vi "Dialog GraphSetting (Wave).vi"(11 "波形グラフref(in)":refnum<vi>) -> ()   [LabVIEW 2014]
uses:
  TypeDef/GraphSetting Appearance.ctl
  TypeDef/GraphSetting Plot.ctl
  SupportVIs/GraphSetting Scale.ctl
  TypeDef/GraphSetting DisplayFormatType.ctl
  TypeDef/GraphSetting All.ctl
  TypeDef/GraphSetting Command.ctl
  Lib/Event/Write User Event (Array).vi
  <vilib>/Utility/xml.llb/Write to XML File(string).vi
  <vilib>/Utility/xml.llb/Read From XML File(string).vi
  <vilib>/measure/NI_MABase.lvlib
panel:
  out "波形グラフ":cluster{dbl, "dt":dbl, "Y":dbl[]}[](graph)
  in  "ファイル読込":bool
  in  "ファイル保存":bool
  in  "タブ制御器":enum32{"外観", "スケール", "プロット"}(tab)
  in  "外観":T1
  in  "Yスケール選択":u16(ring) items=["振幅"]
  in  "スケール(Y軸)":T2
  in  "スケール(X軸)":T2
  in  "Xスケール選択":u16(ring) items=["周波数"]
  in  "プロット":T4 {"Yスケール" items=["振幅"]; "Xスケール" items=["周波数"]; "プロット補間" max=5 step=1; "ポイントスタイル" max=16 step=1; "太さ" max=5 step=1; "ラインスタイル" max=4 step=1}
  in  "プロット選択":u16(ring) items=["プロット0", "プロット1"]
  in  "停止ボタン":bool
  # "スケールのスタイルとカラー"
  # "スケール係数"
  # "スケールのスタイルとカラー"
  # "スケールのスタイルとカラー"
  # "スケール係数"
  # "スケールのスタイルとカラー"
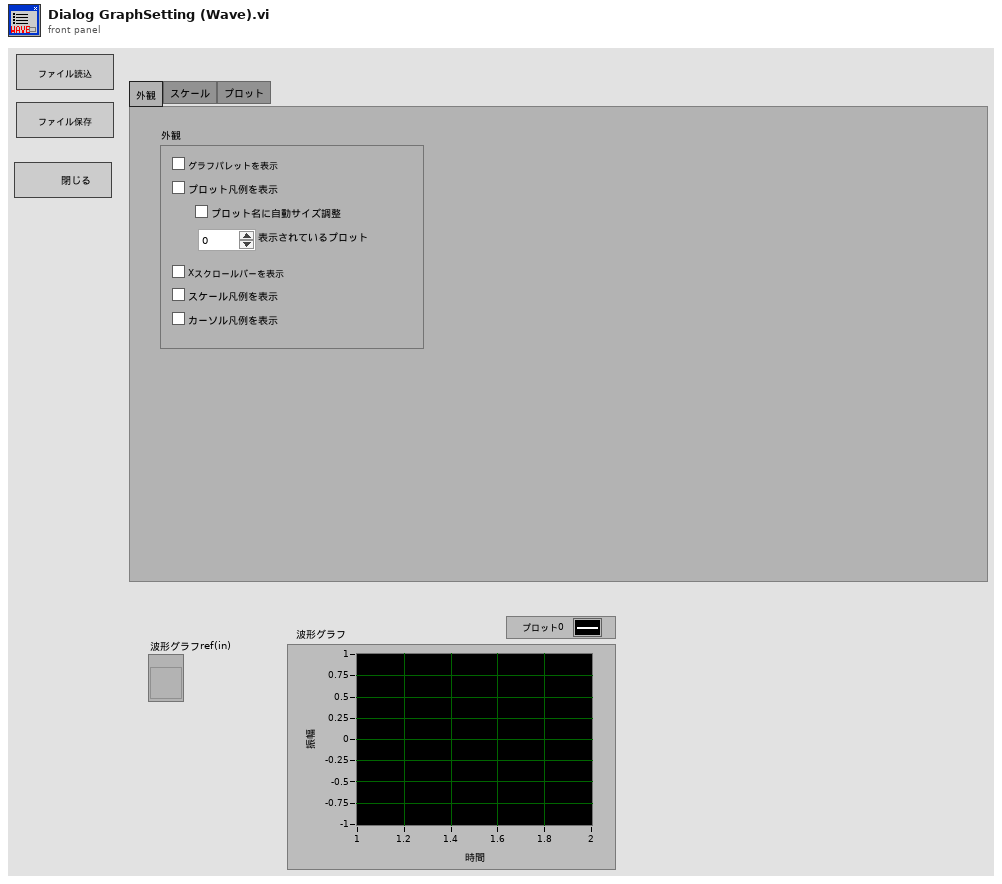
[diagram p1: front panel]
types:
  T1 = typedef "GraphSetting Appearance.ctl" = cluster{"グラフパレットを表示":bool, "プロット凡例を表示":bool, "プロット名に自動サイズ調整":bool, "表示されているプロット":u32, "Xスクロールバーを表示":bool, "スケール凡例を表示":bool, "カーソル凡例を表示":bool}
  T2 = typedef "GraphSetting Scale.ctl" = cluster{"名前":string, "スケールラベルを表示":bool, "スケールを表示":bool, "ログ":bool, "反転":bool, "自動スケール":bool, "最小":dbl, "最大":dbl, "オフセット":dbl, "乗数":dbl, "主目盛り":u32, "補助目盛り":u32, "マーカテキスト":u32, "主グリッド":u32, "補助グリッド":u32, "タイプ":T3, "小数点以下桁数":u8}
  T3 = typedef "GraphSetting DisplayFormatType.ctl" = enum8{"浮動小数点", "科学", "工学", "バイナリ", "８進数", "１６進数", "相対時間", "時間と日時", "SI"}
  T4 = typedef "GraphSetting Plot.ctl" = cluster{"名前":string, "表示":bool, "ラインスタイル":u8, "太さ":u8, "ポイントスタイル":u8, "プロット補間":u8, "ラインカラー":u32, "ポイント/塗りつぶし":u32, "Xスケール":u16, "Yスケール":u16}
  T5 = typedef "GraphSetting All.ctl" = cluster{"外観":T1, "スケールX[]":T2[], "スケールY[]":T2[], "プロット[]":T4[]}
  T6 = typedef "GraphSetting Command.ctl" = enum16{"Get(ref->ctl)", "Set(ctl->ref)"}
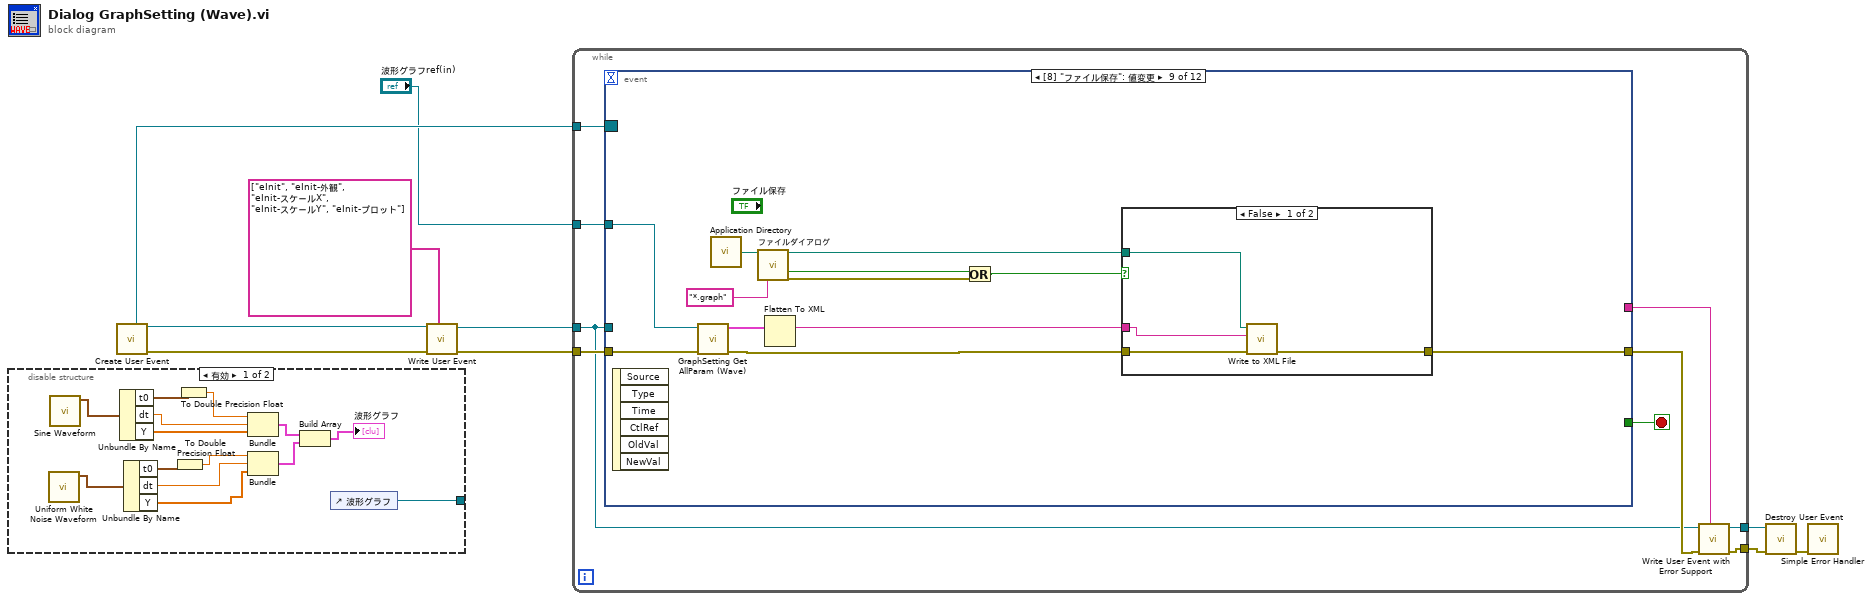
[diagram p0: block diagram]
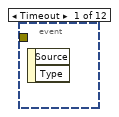
[diagram p3: hidden frame]
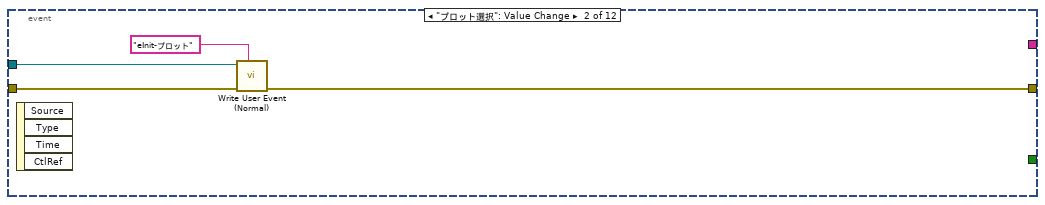
[diagram p4: hidden frame]
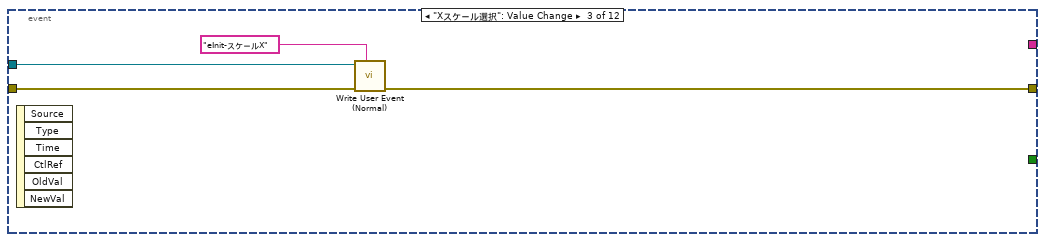
[diagram p5: hidden frame]
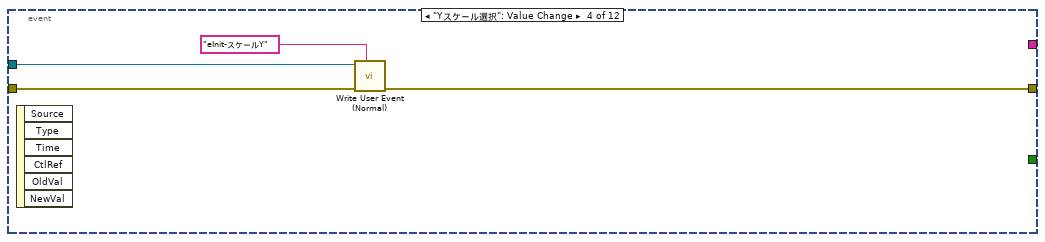
[diagram p6: hidden frame]
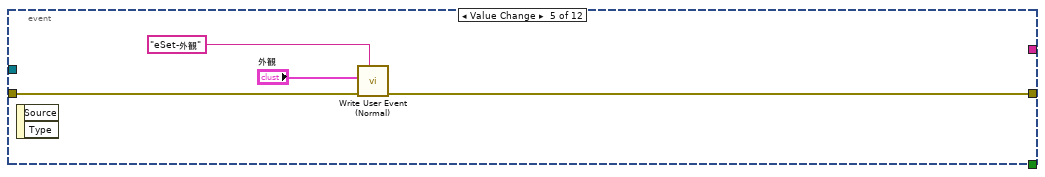
[diagram p7: hidden frame]
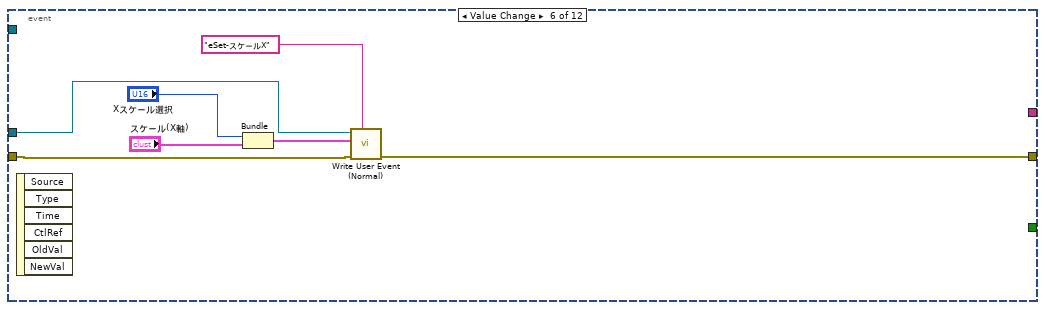
[diagram p8: hidden frame]
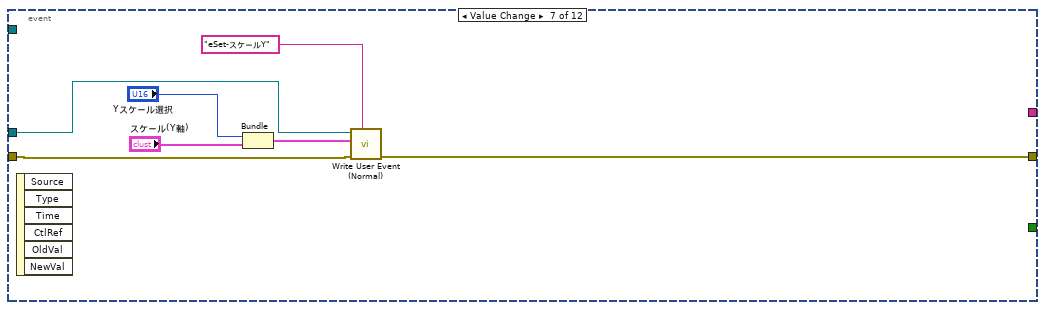
[diagram p9: hidden frame]
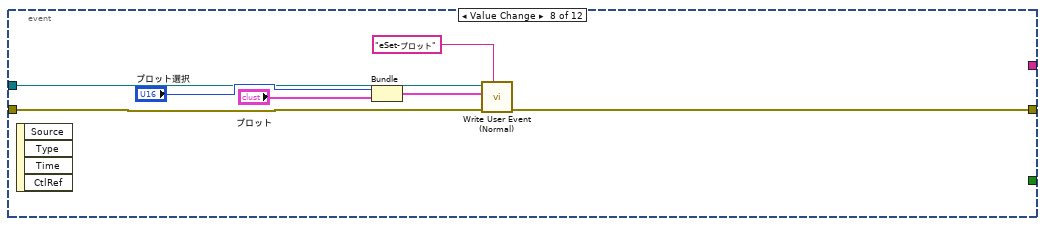
[diagram p10: hidden frame]
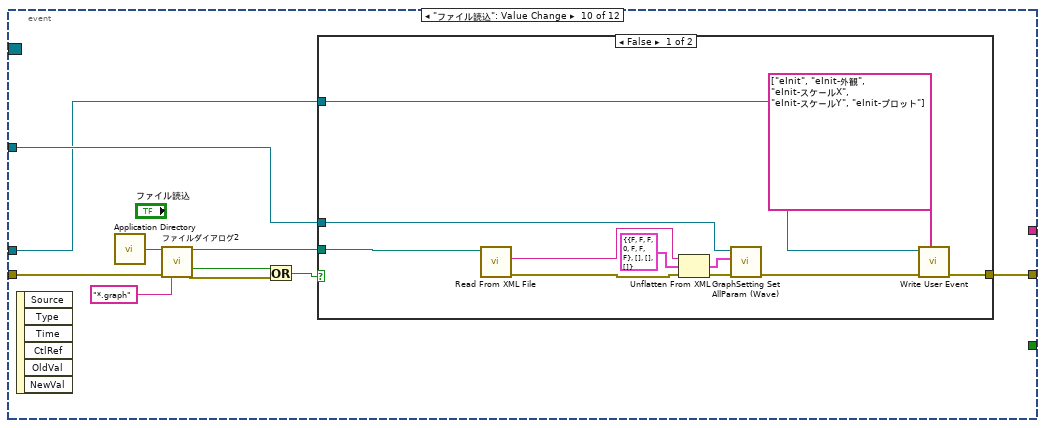
[diagram p12: hidden frame]
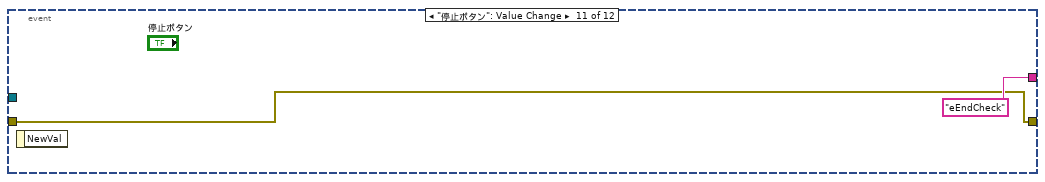
[diagram p14: hidden frame]
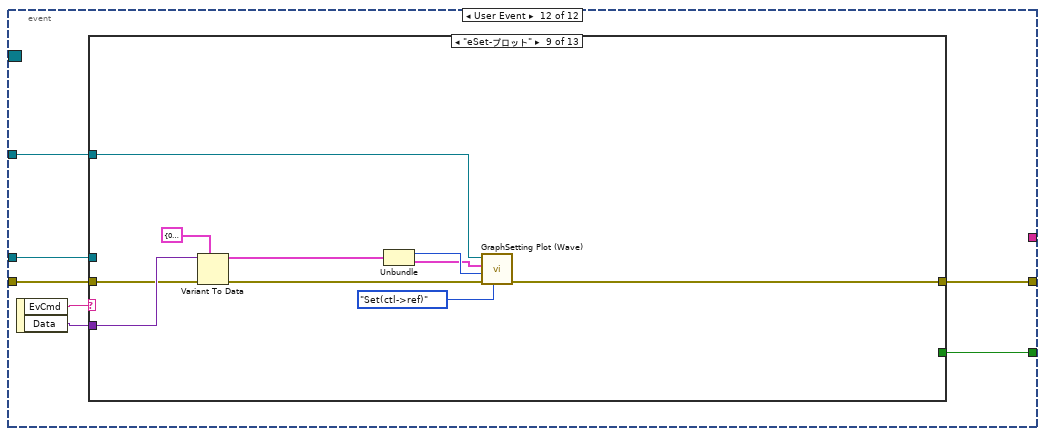
[diagram p15: hidden frame]
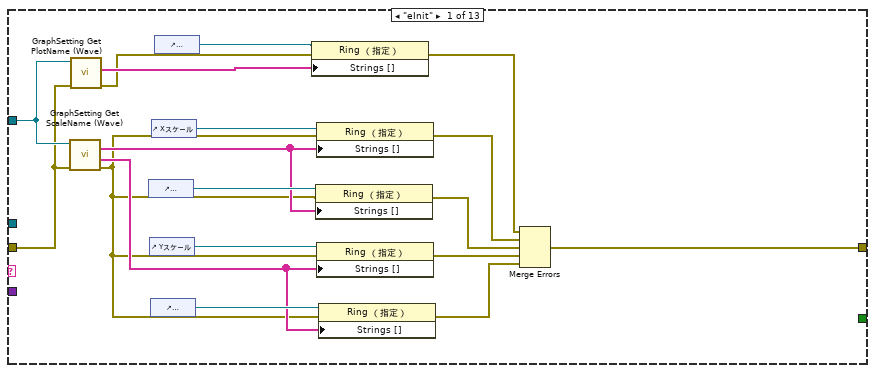
[diagram p16: hidden frame]
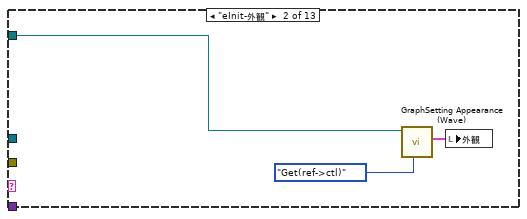
[diagram p17: hidden frame]
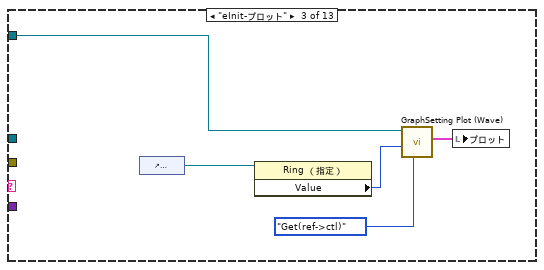
[diagram p18: hidden frame]
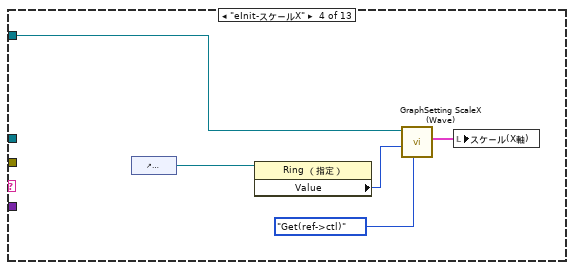
[diagram p19: hidden frame]
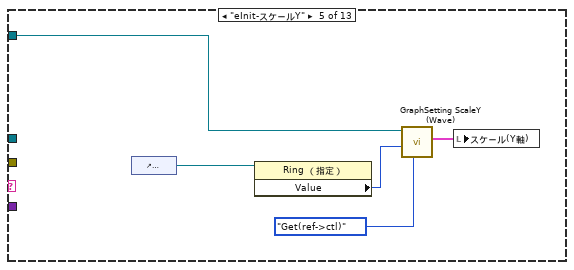
[diagram p20: hidden frame]
diagram:
  n1 = disable-structure shown="有効" {
    disable-tunnel: [w11 _] -> _
    frame Enabled {
      n2 = call <vilib>:"Uniform White Noise Waveform.vi"() -> ("signal out"=w19:waveform(dbl))  [unwired: 10 in, 1 out]
      n3 = call <vilib>:"Sine Waveform.vi"() -> ("signal out"=w24:waveform(dbl))  [unwired: 10 in, 1 out]
      n4 = Unbundle By Name(w24) -> ("t0"=w23:timestamp, "dt"=w21:dbl, "Y"=w20:dbl[])
      n5 = Unbundle By Name(w19) -> ("t0"=w18:timestamp, "dt"=w16:dbl, "Y"=w15:dbl[])
      n6 = To Double Precision Float(number=w18) -> (double precision float=w17:dbl)
      n7 = To Double Precision Float(number=w23) -> (double precision float=w22:dbl)
      n8 = Bundle(w22, "dt"=w21, "Y"=w20) -> (w14:cluster{dbl, "dt":dbl, "Y":dbl[]})  [unwired: 1 in]
      n9 = Bundle(w17, "dt"=w16, "Y"=w15) -> (w13:cluster{dbl, "dt":dbl, "Y":dbl[]})  [unwired: 1 in]
      n10 = Build Array(w14, w13) -> (→"波形グラフ":cluster{dbl, "dt":dbl, "Y":dbl[]}[])
      n11 = control-ref of="波形グラフ"() -> (w11:refnum<vi>)
    }
    frame Disabled {
    }
  }
  n12 = call "Create User Event.vi"() -> ("error out"=w8:errorcluster, "User Event"=w9:refnum<user-event>, "Event Registration Refnum"=w10:refnum<event-registration>)  [unwired: 9 in]
  n13 = call-poly "Write User Event.vi"("EvCmd[]"=string[] ["eInit", "eInit-外観", "eInit-スケールX", "eInit-スケールY", "eInit-プロット"], "エラー入力（エラーなし）"=w8, "ユーザイベント入力"=w9) -> ("エラー出力"=w4:errorcluster, "ユーザイベント出力"=w5:refnum<user-event>)  [unwired: 7 in]
  n14 = while {
    tunnel: w4 -> [w32]
    tunnel: w10 -> [w33]
    tunnel: [w29] -> w7
    tunnel: w5 -> [w25]
    tunnel: "波形グラフref(in)" -> [w31]
    tunnel: [w26] -> w2
    stop <- w27 stop-if-true
    n15 = event shown="[8] \"ファイル保存\": 値変更" {
      selector: w33 -> [_ _ _ _ _ _ _ _ _ _ _ _]
      dyn-events: _ -> [_ _ _ _ _ _ _ _ _ _ _ _]
      timeout: _ -> [_ _ _ _ _ _ _ _ _ _ _ _]
      tunnel: [_ _ _ _ _ _ _ _ _ _ _ w113] -> w27
      tunnel: [_ w35 w39 w42 w46 w51 w58 w65 w78 w91 w109 w114] -> w30
      tunnel: w32 -> [_ w36 w41 w44 w47 w50 w59 w66 w75 w95 w109 w115]
      tunnel: w25 -> [_ w37 w40 w43 _ w54 w60 w67 _ w90 _ w112]
      tunnel: w31 -> [_ _ _ _ _ _ _ _ w74 w92 _ w111]
      tunnel: [_ _ _ _ _ _ _ _ _ _ "eEndCheck" _] -> w28
      event Timeout {
        n16 = event-data() -> ()  [unwired: 1 in, 2 out]
      }
      event "プロット選択": Value Change {
        n17 = event-data() -> ()  [unwired: 1 in, 4 out]
        n18 = call "Write User Event (Normal).vi"("EvCmd"="eInit-プロット", "エラー入力（エラーなし）"=w36, "ユーザイベント入力"=w37) -> ("エラー出力"=w35:errorcluster)  [unwired: 7 in, 1 out]
      }
      event "Xスケール選択": Value Change {
        n19 = event-data() -> ()  [unwired: 1 in, 6 out]
        n20 = call "Write User Event (Normal).vi"("EvCmd"="eInit-スケールX", "エラー入力（エラーなし）"=w41, "ユーザイベント入力"=w40) -> ("エラー出力"=w39:errorcluster)  [unwired: 7 in, 1 out]
      }
      event "Yスケール選択": Value Change {
        n21 = event-data() -> ()  [unwired: 1 in, 6 out]
        n22 = call "Write User Event (Normal).vi"("EvCmd"="eInit-スケールY", "エラー入力（エラーなし）"=w44, "ユーザイベント入力"=w43) -> ("エラー出力"=w42:errorcluster)  [unwired: 7 in, 1 out]
      }
      event Value Change {
        n23 = event-data() -> ()  [unwired: 1 in, 2 out]
        n24 = call "Write User Event (Normal).vi"("EvCmd"="eSet-外観", "エラー入力（エラーなし）"=w47, "データ"="外観") -> ("エラー出力"=w46:errorcluster)  [unwired: 7 in, 1 out]
      }
      event Value Change {
        n25 = event-data() -> ()  [unwired: 1 in, 6 out]
        n26 = Bundle("Xスケール選択"="Xスケール選択", "スケール(X軸)"="スケール(X軸)") -> (w55:cluster{"Xスケール選択":u16, "スケール(X軸)":T2})  [unwired: 1 in]
        n27 = call "Write User Event (Normal).vi"("EvCmd"="eSet-スケールX", "エラー入力（エラーなし）"=w50, "データ"=w55, "ユーザイベント入力"=w54) -> ("エラー出力"=w51:errorcluster)  [unwired: 6 in, 1 out]
      }
      event Value Change {
        n28 = event-data() -> ()  [unwired: 1 in, 6 out]
        n29 = Bundle("Yスケール選択"="Yスケール選択", "スケール(Y軸)"="スケール(Y軸)") -> (w61:cluster{"Yスケール選択":u16, "スケール(Y軸)":T2})  [unwired: 1 in]
        n30 = call "Write User Event (Normal).vi"("EvCmd"="eSet-スケールY", "エラー入力（エラーなし）"=w59, "データ"=w61, "ユーザイベント入力"=w60) -> ("エラー出力"=w58:errorcluster)  [unwired: 6 in, 1 out]
      }
      event Value Change {
        n31 = event-data() -> ()  [unwired: 1 in, 4 out]
        n32 = Bundle("プロット選択"="プロット選択", "プロット"="プロット") -> (w68:cluster{"プロット選択":u16, "プロット":T4})  [unwired: 1 in]
        n33 = call "Write User Event (Normal).vi"("EvCmd"="eSet-プロット", "エラー入力（エラーなし）"=w66, "データ"=w68, "ユーザイベント入力"=w67) -> ("エラー出力"=w65:errorcluster)  [unwired: 6 in, 1 out]
      }
      event "ファイル保存": Value Change {
        n34 = event-data() -> ()  [unwired: 1 in, 6 out]
        n35 = call "GraphSetting Get AllParam (Wave).vi"("エラー入力（エラーなし）"=w75, "波形グラフref(in)"=w74) -> ("エラー出力"=w77:errorcluster, "クラスタ"=w76:cluster{"外観(out)":T1, T2[], T2[], T4[]})  [unwired: 8 in]
        n36 = call <vilib>:"Application Directory.vi"() -> ("Application Directory"=w81:path)
        n37 = call "ファイルダイアログ"("start path"=w81, "pattern (all files)"="*.graph") -> ("selected path"=w79:path, "cancelled"=w72:bool, "error out"=w73:errorcluster)  [unwired: 10 in, 1 out]
        n38 = Flatten To XML(anything=w76) -> (xml string=w80:string)
        n39 = Or(x=w72, y=w73) -> (x .or. y?=w71:bool)
        n40 = case shown="FALSE" w71 {
          tunnel: w79 -> [w86 _]
          tunnel: w80 -> [w85 _]
          tunnel: w77 -> [w83 w87]
          tunnel: [w84 w87] -> w78
          frame False {
            n41 = call-poly <vilib>:"Write to XML File.vi"("error in (no error)"=w83, "XML Input"=w85, "XML File Path"=w86) -> ("error out"=w84:errorcluster)  [unwired: 6 in, 2 out]
          }
          frame True {
          }
        }
      }
      event "ファイル読込": Value Change {
        n42 = event-data() -> ()  [unwired: 1 in, 6 out]
        n43 = call <vilib>:"Application Directory.vi"() -> ("Application Directory"=w97:path)
        n44 = call "ファイルダイアログ2"("start path"=w97, "error in"=w95, "pattern (all files)"="*.graph") -> ("selected path"=w94:path, "cancelled"=w89:bool, "error out"=w88:errorcluster)  [unwired: 9 in, 1 out]
        n45 = Or(x=w89, y=w88) -> (x .or. y?=w93:bool)
        n46 = case shown="FALSE" w93 {
          tunnel: w94 -> [w106 _]
          tunnel: w92 -> [w102 _]
          tunnel: [w99 _] -> w91
          tunnel: w90 -> [w101 _]
          frame False {
            n47 = call-poly <vilib>:"Read From XML File.vi"("XML File Path"=w106) -> ("error out"=w105:errorcluster, "XML Elements"=w107:string)  [unwired: 8 in, 1 out]
            n48 = Unflatten From XML(xml string=w107, type=T5 {"外観"={"グラフパレットを表示"=FALSE, "プロット凡例を表示"=FALSE, "プロット名に自動サイズ調整"=FALSE, "表示されているプロット"=0, "Xスクロールバーを表示"=FALSE, "スケール凡例を表示"=FALSE, "カーソル凡例を表示"=FALSE}, "スケールX[]"=[], "スケールY[]"=[], "プロット[]"=[]} ("出力クラスタ"), error in (no error)=w105) -> (value=w104:T5, error out=w103:errorcluster)
            n49 = call "GraphSetting Set AllParam (Wave).vi"("error in (no error)"=w103, "Chartグラフパラメータ"=w104, "波形グラフref(in)"=w102) -> ("error out"=w100:errorcluster)  [unwired: 8 in]
            n50 = call-poly "Write User Event.vi"("EvCmd[]"=string[] ["eInit", "eInit-外観", "eInit-スケールX", "eInit-スケールY", "eInit-プロット"], "エラー入力（エラーなし）"=w100, "ユーザイベント入力"=w101) -> ("エラー出力"=w99:errorcluster)  [unwired: 7 in, 1 out]
          }
          frame True {
          }
        }
      }
      event "停止ボタン": Value Change {
        n51 = event-data() -> ()  [unwired: 1 in, 1 out]
      }
      event User Event {
        n52 = event-data() -> ("EvCmd"=w117:string, "Data"=w116:variant)  [unwired: 1 in]
        n53 = case shown="\"eSet-プロット\"" w117 {
          selector: w117 -> [_ _ _ _ _ _ _ _ _ _ _ _ w201]
          tunnel: w116 -> [_ _ _ _ _ w158 w166 w177 w187 _ _ w200 _]
          tunnel: w115 -> [w127 _ _ _ _ w156 w168 w176 w186 w191 w195 w198 _]
          tunnel: [w118 _ _ _ _ w154 w161 w170 w180 w190 w195 _ _] -> w114
          tunnel: [_ _ _ _ _ _ _ _ _ _ TRUE TRUE _] -> w113
          tunnel: w112 -> [_ _ _ _ _ _ _ _ _ w193 _ _ _]
          tunnel: w111 -> [w130 w138 w143 w148 w153 w159 w162 w174 w184 _ _ _ _]
          frame "eInit" {
            n54 = call "GraphSetting Get ScaleName (Wave).vi"("error in (no error)"=w127, "波形グラフref(in)"=w130) -> ("error out"=w124:errorcluster, "Y軸名称[]"=w126:string[], "X軸名称[]"=w133:string[])  [unwired: 7 in]
            n55 = call "GraphSetting Get PlotName (Wave).vi"("error in (no error)"=w127, "波形グラフref(in)"=w130) -> ("error out"=w125:errorcluster, "プロット名称[]"=w128:string[])  [unwired: 8 in]
            n56 = control-ref of="Xスケール選択"() -> (w134:refnum<vi>)
            n57 = control-ref of="Yスケール"() -> (w131:refnum<vi>)
            n58 = control-ref of="Yスケール選択"() -> (w132:refnum<vi>)
            n59 = control-ref of="Xスケール"() -> (w135:refnum<vi>)
            n60 = control-ref of="プロット選択"() -> (w129:refnum<vi>)
            n61 = property class="Ring （指定）"(reference=w129, error in=w125, "Strings []"=w128) -> (error out=w123:errorcluster)  [unwired: 1 out]
            n62 = property class="Ring （指定）"(reference=w134, error in=w124, "Strings []"=w133) -> (error out=w121:errorcluster)  [unwired: 1 out]
            n63 = property class="Ring （指定）"(reference=w135, error in=w124, "Strings []"=w133) -> (error out=w122:errorcluster)  [unwired: 1 out]
            n64 = property class="Ring （指定）"(reference=w131, error in=w124, "Strings []"=w126) -> (error out=w120:errorcluster)  [unwired: 1 out]
            n65 = property class="Ring （指定）"(reference=w132, error in=w124, "Strings []"=w126) -> (error out=w119:errorcluster)  [unwired: 1 out]
            n66 = Merge Errors(w123, w122, w121, w120, w119) -> (w118:errorcluster)
          }
          frame "eInit-外観" {
            n67 = call "GraphSetting Appearance (Wave).vi"("コマンド"=GraphSetting_Command."Get(ref->ctl)", "波形グラフref(in)"=w138) -> ("外観(out)"=w137:T1)  [unwired: 8 in, 1 out]
            n68 = local write "外観"(w137) -> ()
          }
          frame "eInit-プロット" {
            n69 = control-ref of="プロット選択"() -> (w142:refnum<vi>)
            n70 = property class="Ring （指定）"(reference=w142) -> ("Value"=w141:u16)  [unwired: 1 in, 2 out]
            n71 = call "GraphSetting Plot (Wave).vi"("コマンド"=GraphSetting_Command."Get(ref->ctl)", "アクティブプロット"=w141, "波形グラフref(in)"=w143) -> ("プロット(out)"=w139:T4)  [unwired: 7 in, 1 out]
            n72 = local write "プロット"(w139) -> ()
          }
          frame "eInit-スケールX" {
            n73 = control-ref of="Xスケール選択"() -> (w147:refnum<vi>)
            n74 = property class="Ring （指定）"(reference=w147) -> ("Value"=w146:u16)  [unwired: 1 in, 2 out]
            n75 = call "GraphSetting ScaleX (Wave).vi"("コマンド"=GraphSetting_Command."Get(ref->ctl)", "アクティブスケール(X)"=w146, "波形グラフref(in)"=w148) -> ("スケール(out)"=w144:T2)  [unwired: 7 in, 1 out]
            n76 = local write "スケール(X軸)"(w144) -> ()
          }
          frame "eInit-スケールY" {
            n77 = control-ref of="Yスケール選択"() -> (w152:refnum<vi>)
            n78 = property class="Ring （指定）"(reference=w152) -> ("Value"=w151:u16)  [unwired: 1 in, 2 out]
            n79 = call "GraphSetting ScaleY (Wave).vi"("コマンド"=GraphSetting_Command."Get(ref->ctl)", "アクティブスケールY"=w151, "波形グラフref(in)"=w153) -> ("スケール(out)"=w149:T2)  [unwired: 7 in, 1 out]
            n80 = local write "スケール(Y軸)"(w149) -> ()
          }
          frame "eSet-外観" {
            n81 = Variant To Data(error in=w156, Variant=w158) -> (data=w157:T1, error out=w155:errorcluster)  [unwired: 1 in]
            n82 = call "GraphSetting Appearance (Wave).vi"("コマンド"=GraphSetting_Command."Set(ctl->ref)", "error in (no error)"=w155, "外観(in)"=w157, "波形グラフref(in)"=w159) -> ("error out"=w154:errorcluster)  [unwired: 6 in, 1 out]
          }
          frame "eSet-スケールX" {
            n83 = Variant To Data(type=cluster{"Xスケール選択":u16, "スケール(X軸)":T2} {"Xスケール選択"=0, "スケール(X軸)"={"名前"="", "スケールラベルを表示"=FALSE, "スケールを表示"=FALSE, "ログ"=FALSE, "反転"=FALSE, "自動スケール"=FALSE, "最小"=0.0, "最大"=0.0, "オフセット"=0.0, "乗数"=0.0, "主目盛り"=0, "補助目盛り"=0, "マーカテキスト"=0, "主グリッド"=0, "補助グリッド"=0, "タイプ"=enum."浮動小数点", "小数点以下桁数"=0}} ("出力クラスタ"), Variant=w166) -> (data=w165:cluster{"Xスケール選択":u16, "スケール(X軸)":T2})  [unwired: 1 in, 1 out]
            n84 = Unbundle(w165) -> ("Xスケール選択"=w163:u16, "スケール(X軸)"=w164:T2)
            n85 = call "GraphSetting ScaleX (Wave).vi"("コマンド"=GraphSetting_Command."Set(ctl->ref)", "error in (no error)"=w168, "アクティブスケール(X)"=w163, "スケール(in)"=w164, "波形グラフref(in)"=w162) -> ("error out"=w161:errorcluster)  [unwired: 5 in, 1 out]
          }
          frame "eSet-スケールY" {
            n86 = Variant To Data(error in=w176, type=cluster{"Xスケール選択":u16, "スケール(X軸)":T2} {"Xスケール選択"=0, "スケール(X軸)"={"名前"="", "スケールラベルを表示"=FALSE, "スケールを表示"=FALSE, "ログ"=FALSE, "反転"=FALSE, "自動スケール"=FALSE, "最小"=0.0, "最大"=0.0, "オフセット"=0.0, "乗数"=0.0, "主目盛り"=0, "補助目盛り"=0, "マーカテキスト"=0, "主グリッド"=0, "補助グリッド"=0, "タイプ"=enum."浮動小数点", "小数点以下桁数"=0}} ("出力クラスタ"), Variant=w177) -> (data=w175:cluster{"Xスケール選択":u16, "スケール(X軸)":T2}, error out=w171:errorcluster)
            n87 = Unbundle(w175) -> ("Xスケール選択"=w172:u16, "スケール(X軸)"=w173:T2)
            n88 = call "GraphSetting ScaleY (Wave).vi"("コマンド"=GraphSetting_Command."Set(ctl->ref)", "error in (no error)"=w171, "アクティブスケールY"=w172, "スケール(in)"=w173, "波形グラフref(in)"=w174) -> ("error out"=w170:errorcluster)  [unwired: 5 in, 1 out]
          }
          frame "eSet-プロット" {
            n89 = Variant To Data(error in=w186, type=cluster{"プロット選択":u16, "プロット":T4} {"プロット選択"=0, "プロット"={"名前"="", "表示"=FALSE, "ラインスタイル"=0, "太さ"=0, "ポイントスタイル"=0, "プロット補間"=0, "ラインカラー"=0, "ポイント/塗りつぶし"=0, "Xスケール"=0, "Yスケール"=0}} ("出力クラスタ"), Variant=w187) -> (data=w185:cluster{"プロット選択":u16, "プロット":T4}, error out=w183:errorcluster)
            n90 = Unbundle(w185) -> ("プロット選択"=w182:u16, "プロット"=w181:T4)
            n91 = call "GraphSetting Plot (Wave).vi"("コマンド"=GraphSetting_Command."Set(ctl->ref)", "error in (no error)"=w183, "アクティブプロット"=w182, "プロット(in)"=w181, "波形グラフref(in)"=w184) -> ("error out"=w180:errorcluster)  [unwired: 5 in, 1 out]
          }
          frame "eEndCheck" {
            n92 = call "Write User Event (Normal).vi"("EvCmd"="eNormalEnd", "エラー入力（エラーなし）"=w191, "ユーザイベント入力"=w193) -> ("エラー出力"=w190:errorcluster)  [unwired: 7 in, 1 out]
          }
          frame "eNormalEnd" {
          }
          frame "eErrorEnd" {
            n93 = Variant To Data(error in=w198, type=errorcluster {"status"=FALSE, "code"=0, "source"=""} ("エラー定数"), Variant=w200) -> (data=w197:errorcluster)  [unwired: 1 out]
            n94 = call <vilib>:"Simple Error Handler.vi"("error in (no error)"=w197) -> ()  [unwired: 4 in, 5 out]
          }
          frame Default {
            n95 = call "DialogProgramError.vi"("エラー内容"="ユーザイベント例外" ("エラー詳細"), "エラー詳細"=w201) -> ()  [unwired: 9 in, 1 out]
          }
        }
      }
    }
    n96 = call "Write User Event with Error Support.vi"("EvCmd"=w28, "エラー入力（エラーなし）"=w30, "ユーザイベント入力"=w25) -> ("エラー出力"=w29:errorcluster, "ユーザイベント出力"=w26:refnum<user-event>)  [unwired: 7 in]
  }
  n97 = call "Destroy User Event.vi"("error in (no error)"=w7, "User Event"=w2) -> ("error out"=w6:errorcluster)  [unwired: 9 in]
  n98 = call <vilib>:"Simple Error Handler.vi"("error in (no error)"=w6) -> ()  [unwired: 4 in, 5 out]
